vi "FeedbackDecode.vi"() -> ()   [LabVIEW 2020] (continued)
            n1857 = Cluster To Array(cluster=w1907) -> (array=w1906:bool[])
            n1858 = local read "DecodeClust"() -> (w1905:T5)
            n1859 = Boolean Array To Number(Boolean array=w1906) -> (number=w1904:u32)
            n1860 = local read "UEAHMIdx"() -> (w1924:i32[])
            n1861 = call "FeedbackDecode_PlotHeatmap.vi"("MousePos"=w1910, "Instance"=1, "Mode"=w1912) -> ("CurrPos"=w1923:i32)  [unwired: 3 in, 1 out]
            n1862 = call "FeedbackDecode_PlotHeatmap.vi"("MousePos"=w1911, "Instance"=0, "Mode"=w1912) -> ()  [unwired: 3 in, 2 out]
            n1863 = call "FeedbackDecode_PlotHeatmap.vi"("MousePos"=w1911, "Instance"=2, "Mode"=w1912) -> ()  [unwired: 3 in, 2 out]
            n1864 = Search 1D Array(1D array=w1924, element=w1923) -> (index of element=w1909:i32)  [unwired: 1 in]
            n1865 = Add(x=w1909, y=101) -> (x+y=w1903:i32)
            n1866 = case shown="4" w1904 {
              tunnel: w1903 -> [_ w1928 w1932]
              tunnel: w1905 -> [w1925 w1927 w1931]
              tunnel: [w1925 w1926 w1930] -> w1902
              frame 0, Default {
              }
              frame 18 {
                # "ctrl"
                n1867 = call "FeedbackDecode_UpdateDecodeClustElect.vi"("DecodeClustIn"=w1927, "KalmanElect"=w1928) -> ("DecodeClustOut"=w1926:T5)  [unwired: 1 in]
              }
              frame 4 {
                # "alt"
                n1868 = Unbundle By Name(w1931) -> ("BadUEAElects"=w1933:dbl[])
                n1869 = Insert Into Array(array=w1933, new element=w1932) -> (w1929:dbl[])  [unwired: 1 in]
                n1870 = Bundle By Name(cluster=w1931, "BadUEAElects"=w1929) -> (w1930:T5)
                n1871 = property on="BadUEAElects" class="Arr (strict)"("Val(Sgnl)"=w1929) -> ()  [unwired: 2 in, 2 out]
              }
            }
            n1872 = local read "LoopCnt"() -> (w1917:u64)
            n1873 = call-poly "FeedbackDecode_VariablesToString.vi"("Format"="%0.0f", "ValueIn"=w1903, "FieldName"="SelElect") -> ("StringOut"=w1919:string)  [unwired: 4 in]
            n1874 = local write "SelElect"(w1903) -> ()
            n1875 = local write "BaseCnt2"(w1917) -> ()
            n1876 = Bundle By Name(cluster=w1902, "ClearWfs"=TRUE, "SelElect"=w1903, "EventStr"=w1919) -> (w1901:T5)
            n1877 = call "FeedbackDecode_MLComCtrl.vi"("DecodeClustIn"=w1901, "Mode"=T19."SendEvent") -> ("DecodeClustOut"=w1900:T5)  [unwired: 6 in, 3 out]
            n1878 = local write "DecodeClust"(w1900) -> ()
          }
          event "EMGHM": Mouse Down {
            w1945 = cluster{"X":i32, "Y":i32} {"X"=0, "Y"=0} ("MousePos")
            w1946 = enum16{"Initialize", "Run", "Mouse"}."Mouse" ("Mode")
            n1879 = event-data() -> ("PlatMods"=w1942:T51, "Coords"=w1944:T45)  [unwired: 1 in, 4 out]
            n1880 = local read "DecodeClust"() -> (w1939:T5)
            n1881 = Cluster To Array(cluster=w1942) -> (array=w1941:bool[])
            n1882 = Boolean Array To Number(Boolean array=w1941) -> (number=w1940:u32)
            n1883 = local read "EMGHMIdx"() -> (w1958:i32[])
            n1884 = call "FeedbackDecode_PlotHeatmap.vi"("MousePos"=w1944, "Instance"=2, "Mode"=w1946) -> ("CurrPos"=w1957:i32)  [unwired: 3 in, 1 out]
            n1885 = call "FeedbackDecode_PlotHeatmap.vi"("MousePos"=w1945, "Instance"=0, "Mode"=w1946) -> ()  [unwired: 3 in, 2 out]
            n1886 = call "FeedbackDecode_PlotHeatmap.vi"("MousePos"=w1945, "Instance"=1, "Mode"=w1946) -> ()  [unwired: 3 in, 2 out]
            n1887 = Search 1D Array(1D array=w1958, element=w1957) -> (index of element=w1936:i32)  [unwired: 1 in]
            n1888 = Add(x=w1936, y=201) -> (x+y=w1938:i32)
            n1889 = case shown="4" w1940 {
              tunnel: w1938 -> [_ w1962 _]
              tunnel: w1939 -> [w1959 w1961 w1967]
              tunnel: [w1959 w1960 w1968] -> w1937
              tunnel: w1936 -> [_ _ w1969]
              frame 0, Default {
              }
              frame 18 {
                # "ctrl"
                n1890 = call "FeedbackDecode_UpdateDecodeClustElect.vi"("DecodeClustIn"=w1961, "KalmanElect"=w1962) -> ("DecodeClustOut"=w1960:T5)  [unwired: 1 in]
              }
              frame 4 {
                # "alt"
                n1891 = Quotient & Remainder(x=w1969, y=10.0) -> (x-y*floor(x/y)=w1973:dbl, floor(x/y)=w1975:dbl)
                n1892 = Increment(x=w1973) -> (x+1=w1974:dbl)
                n1893 = Multiply(x=w1975, y=4.0) -> (x*y=w1972:dbl)
                n1894 = Add(x=w1974, y=w1972) -> (x+y=w1963:dbl)
                n1895 = In Range and Coerce(upper limit=32.0, x=w1963, lower limit=1.0) -> (In Range?=w1964:bool)  [unwired: 1 out]
                n1896 = case shown="True" w1964 {
                  tunnel: w1963 -> [_ w1980]
                  tunnel: [w1976 w1979] -> w1968
                  tunnel: w1967 -> [w1976 w1977]
                  frame False {
                  }
                  frame True {
                    n1897 = Unbundle By Name(w1977) -> ("BadEMGChans"=w1981:dbl[])
                    n1898 = Insert Into Array(array=w1981, new element=w1980) -> (w1978:dbl[])  [unwired: 1 in]
                    n1899 = Bundle By Name(cluster=w1977, "BadEMGChans"=w1978) -> (w1979:T5)
                    n1900 = property on="BadEMGChans" class="Arr (strict)"("Val(Sgnl)"=w1978) -> ()  [unwired: 2 in, 2 out]
                  }
                }
              }
            }
            n1901 = call-poly "FeedbackDecode_VariablesToString.vi"("Format"="%0.0f", "ValueIn"=w1938, "FieldName"="SelElect") -> ("StringOut"=w1953:string)  [unwired: 4 in]
            n1902 = local write "SelElect"(w1938) -> ()
            n1903 = Bundle By Name(cluster=w1937, "ClearWfs"=TRUE, "SelElect"=w1938, "EventStr"=w1953) -> (w1934:T5)
            n1904 = local read "LoopCnt"() -> (w1951:u64)
            n1905 = call "FeedbackDecode_MLComCtrl.vi"("DecodeClustIn"=w1934, "Mode"=T19."SendEvent") -> ("DecodeClustOut"=w1935:T5)  [unwired: 6 in, 3 out]
            n1906 = local write "DecodeClust"(w1935) -> ()
            n1907 = local write "BaseCnt2"(w1951) -> ()
          }
          event Value Change {
            n1908 = event-data() -> ()  [unwired: 1 in, 6 out]
            n1909 = local read "EncodeClust"() -> (w1983:T9)
            n1910 = call "File Dialog2"("pattern (all files)"="StimParams*.txt") -> ("selected path"=w1986:path, "exists"=w1990:bool, "cancelled"=w1989:bool)  [unwired: 11 in, 1 out]
            n1911 = Unbundle By Name(w1983) -> ("SelPreset"=w1985:bool[], "Sel"=w1984:bool[])
            n1912 = local read "DecodeClust"() -> (w1982:T5)
            n1913 = Not(x=w1989) -> (.not. x?=w1991:bool)
            n1914 = And(x=w1990, y=w1991) -> (x .and. y?=w1987:bool)
            n1915 = case shown="True" w1987 {
              tunnel: w1986 -> [_ w2021]
              tunnel: w1985 -> [_ w2024]
              tunnel: w1984 -> [_ w2023]
              tunnel: w1983 -> [w1994 w2022]
              tunnel: w1982 -> [_ w2007]
              frame False {
                n1916 = Bundle By Name(cluster=w1994, "AdjClust.LoadTable"=FALSE) -> (w1993:T9)
                n1917 = local write "EncodeClust"(w1993) -> ()
              }
              frame True {
                n1918 = call-poly <vilib>:"Read Delimited Spreadsheet.vi"("file path (dialog if empty)"=w2021) -> ("all rows"=w2025:string[][])  [unwired: 9 in, 5 out]
                n1919 = Array Size(array=w2024) -> (size(s)=w2027:i32)
                n1920 = Array Size(array=w2023) -> (size(s)=w2030:i32)
                n1921 = Initialize Array(FALSE, w2027) -> (w2031:bool[])
                n1922 = Initialize Array(FALSE, w2030) -> (w2032:bool[])
                n1923 = Bundle By Name(cluster=w2022, "SelPreset"=w2031, "Sel"=w2032, "ParamsTable"=w2025, "AdjClust.LoadTable"=FALSE) -> (w2019:T9)
                n1924 = Path To String(path=w2021) -> (string=w2017:string)
                n1925 = call "FeedbackDecode_UpdateParamsTable.vi"("StimClustIn"=w2019) -> ("StimClustOut"=w2020:T9)  [unwired: 2 in]
                n1926 = call "FeedbackDecode_Params2UEA.vi"("StimClustIn"=w2020) -> ("StimClustOut"=w2002:T9)  [unwired: 2 in]
                n1927 = local read "LoopCnt"() -> (w2011:u64)
                n1928 = local read "NIPTime"() -> (w2000:dbl)
                n1929 = call "FeedbackDecode_BuildStimCmd.vi"("EncodeClustIn"=w2002) -> ("EncodeClustOut"=w2001:T9, "StimCmd"=w1996:string)  [unwired: 1 in]
                n1930 = Search and Replace String(input string=w2017, search string=":", replace string="@" ("replace string (\"\")")) -> (result string=w2004:string)  [unwired: 5 in, 3 out]
                n1931 = Format Into String(w2011) -> (resulting string=w2008:string)  [unwired: 3 in, 1 out]
                n1932 = call-poly "FeedbackDecode_VariablesToString.vi"("Format"="%0.0f", "ValueIn"=w2000, "FieldName"="NIPTime" ("Key Word")) -> ("StringOut"=w1997:string)  [unwired: 4 in]
                n1933 = local write "EncodeClust"(w2001) -> ()
                n1934 = Concatenate Strings("LoadStimParams:SS.EventID=" ("string"), w2008) -> (w2010:string)
                n1935 = Concatenate Strings(w2010, ";", "SS.StimParamsFile='" ("string"), w2004, "';" ("string"), w1996, w1997) -> (w2006:string)
                n1936 = local write "StimCmd"(w1996) -> ()
                n1937 = Bundle By Name(cluster=w2007, "EventStr"=w2006) -> (w2009:T5)
                n1938 = local read "EventParamsFID"() -> (w2015:refnum<file>)
                n1939 = call "FeedbackDecode_MLComCtrl.vi"("DecodeClustIn"=w2009, "Mode"=T19."SendEvent") -> ()  [unwired: 6 in, 4 out]
                n1940 = call "FeedbackDecode_WriteTextEOL.vi"("text"=w2006, "refnum in"=w2015) -> ()  [unwired: 8 in, 2 out]
              }
            }
          }
          event Value Change {
            n1941 = event-data() -> ()  [unwired: 1 in, 6 out]
            n1942 = local read "EncodeClust"() -> (w2034:T9)
            n1943 = call "File Dialog3"("pattern (all files)"="StimPresets*.txt") -> ("selected path"=w2037:path, "exists"=w2041:bool, "cancelled"=w2040:bool)  [unwired: 11 in, 1 out]
            n1944 = Unbundle By Name(w2034) -> ("SelPreset"=w2036:bool[], "Sel"=w2035:bool[])
            n1945 = local read "DecodeClust"() -> (w2033:T5)
            n1946 = Not(x=w2040) -> (.not. x?=w2042:bool)
            n1947 = And(x=w2041, y=w2042) -> (x .and. y?=w2038:bool)
            n1948 = case shown="True" w2038 {
              tunnel: w2037 -> [_ w2073]
              tunnel: w2036 -> [_ w2076]
              tunnel: w2035 -> [_ w2075]
              tunnel: w2034 -> [w2045 w2074]
              tunnel: w2033 -> [_ w2060]
              frame False {
                n1949 = Bundle By Name(cluster=w2045, "AdjClust.LoadTable"=FALSE) -> (w2044:T9)
                n1950 = local write "EncodeClust"(w2044) -> ()
              }
              frame True {
                n1951 = call-poly <vilib>:"Read Delimited Spreadsheet.vi"("file path (dialog if empty)"=w2073) -> ("all rows"=w2077:string[][])  [unwired: 9 in, 5 out]
                n1952 = Array Size(array=w2076) -> (size(s)=w2079:i32)
                n1953 = Array Size(array=w2075) -> (size(s)=w2082:i32)
                n1954 = Initialize Array(FALSE, w2079) -> (w2083:bool[])
                n1955 = Initialize Array(FALSE, w2082) -> (w2084:bool[])
                n1956 = Bundle By Name(cluster=w2074, "SelPreset"=w2083, "Sel"=w2084, "PresetTable"=w2077, "PresetClust.Load"=FALSE ("AdjClust.LoadTable")) -> (w2048:T9)
                n1957 = Path To String(path=w2073) -> (string=w2070:string)
                n1958 = call "FeedbackDecode_UpdatePresetsTable.vi"("StimClustIn"=w2048) -> ("StimClustOut"=w2047:T9)  [unwired: 2 in]
                n1959 = call "FeedbackDecode_UpdateParamsTable.vi"("StimClustIn"=w2047) -> ("StimClustOut"=w2072:T9)  [unwired: 2 in]
                n1960 = call "FeedbackDecode_Params2UEA.vi"("StimClustIn"=w2072) -> ("StimClustOut"=w2055:T9)  [unwired: 2 in]
                n1961 = local read "LoopCnt"() -> (w2064:u64)
                n1962 = local read "NIPTime"() -> (w2053:dbl)
                n1963 = call "FeedbackDecode_BuildStimCmd.vi"("EncodeClustIn"=w2055) -> ("EncodeClustOut"=w2054:T9, "StimCmd"=w2049:string)  [unwired: 1 in]
                n1964 = Search and Replace String(input string=w2070, search string=":", replace string="@" ("replace string (\"\")")) -> (result string=w2057:string)  [unwired: 5 in, 3 out]
                n1965 = Format Into String(w2064) -> (resulting string=w2061:string)  [unwired: 3 in, 1 out]
                n1966 = call-poly "FeedbackDecode_VariablesToString.vi"("Format"="%0.0f", "ValueIn"=w2053, "FieldName"="NIPTime" ("Key Word")) -> ("StringOut"=w2050:string)  [unwired: 4 in]
                n1967 = local write "EncodeClust"(w2054) -> ()
                n1968 = Concatenate Strings("LoadPresets:SS.EventID=" ("string"), w2061) -> (w2063:string)
                n1969 = Concatenate Strings(w2063, ";", "SS.PresetsFile='" ("string"), w2057, "';" ("string"), w2049, w2050) -> (w2059:string)
                n1970 = local write "StimCmd"(w2049) -> ()
                n1971 = Bundle By Name(cluster=w2060, "EventStr"=w2059) -> (w2062:T5)
                n1972 = local read "EventParamsFID"() -> (w2068:refnum<file>)
                n1973 = call "FeedbackDecode_MLComCtrl.vi"("DecodeClustIn"=w2062, "Mode"=T19."SendEvent") -> ()  [unwired: 6 in, 4 out]
                n1974 = call "FeedbackDecode_WriteTextEOL.vi"("text"=w2059, "refnum in"=w2068) -> ()  [unwired: 8 in, 2 out]
              }
            }
          }
          event Value Change {
            n1975 = event-data() -> ()  [unwired: 1 in, 6 out]
            n1976 = local read "DataPath"() -> (w2089:path)
            n1977 = call "File Dialog"("start path"=w2089) -> ("selected path"=w2086:path, "cancelled"=w2088:bool)  [unwired: 11 in, 2 out]
            n1978 = local read "EncodeClust"() -> (w2087:T9)
            n1979 = local read "DecodeClust"() -> (w2085:T5)
            n1980 = case shown="False" w2088 {
              tunnel: w2087 -> [w2100 w2127]
              tunnel: w2086 -> [w2101 _]
              tunnel: w2085 -> [w2091 _]
              frame False {
                w2110 = "_" ("string")
                n1981 = Strip Path(path=w2101) -> (stripped path=w2108:path, name=w2109:string)
                n1982 = Unbundle By Name(w2091) -> ("DataFolder"=w2098:string)
                n1983 = Get Date/Time In Seconds() -> (seconds since 1Jan1904=w2104:timestamp)
                n1984 = Format Date/Time String(time format string (%c)="%H%M%S", seconds (now)=w2104) -> (date/time string=w2106:string)  [unwired: 1 in]
                n1985 = Concatenate Strings("StimParams_" ("name or relative path"), w2098, w2110, w2109, w2110, w2106, ".txt" ("string")) -> (w2107:string)
                n1986 = Unbundle By Name(w2100) -> ("ParamsTable"=w2102:string[][])
                n1987 = Bundle By Name(cluster=w2100, "AdjClust.SaveTable"=FALSE ("Save")) -> (w2120:T9)
                n1988 = Build Path(base path=w2108, name or relative path=w2107) -> (appended path=w2111:path)
                n1989 = call-poly <vilib>:"Write Delimited Spreadsheet.vi"("file path (dialog if empty)"=w2111, "2D data"=w2102) -> ()  [unwired: 12 in, 2 out]
                n1990 = Path To String(path=w2111) -> (string=w2095:string)
                n1991 = local read "LoopCnt"() -> (w2123:u64)
                n1992 = local write "EncodeClust"(w2120) -> ()
                n1993 = Format Into String(w2123) -> (resulting string=w2112:string)  [unwired: 3 in, 1 out]
                n1994 = Search and Replace String(input string=w2095, search string=":", replace string="@" ("replace string (\"\")")) -> (result string=w2093:string)  [unwired: 5 in, 3 out]
                n1995 = local read "NIPTime"() -> (w2117:dbl)
                n1996 = Concatenate Strings("SaveStimParams:SS.EventID=" ("string"), w2112, ";") -> (w2118:string)
                n1997 = local read "EventParamsFID"() -> (w2126:refnum<file>)
                n1998 = call-poly "FeedbackDecode_VariablesToString.vi"("Format"="%0.0f", "ValueIn"=w2117, "FieldName"="NIPTime" ("Key Word")) -> ("StringOut"=w2114:string)  [unwired: 4 in]
                n1999 = Concatenate Strings(w2118, "SS.StimParamsFile='" ("string"), w2093, "';" ("string"), w2114) -> (w2113:string)
                n2000 = call "FeedbackDecode_WriteTextEOL.vi"("text"=w2113, "refnum in"=w2126) -> ()  [unwired: 8 in, 2 out]
                n2001 = Bundle By Name(cluster=w2091, "EventStr"=w2113) -> (w2122:T5)
                n2002 = call "FeedbackDecode_MLComCtrl.vi"("DecodeClustIn"=w2122, "Mode"=T19."SendEvent") -> ()  [unwired: 6 in, 4 out]
              }
              frame True {
                n2003 = Bundle By Name(cluster=w2127, "AdjClust.SaveTable"=FALSE ("Save")) -> (w2129:T9)
                n2004 = local write "EncodeClust"(w2129) -> ()
              }
            }
          }
          event Value Change {
            n2005 = event-data() -> ()  [unwired: 1 in, 6 out]
            n2006 = local read "DataPath"() -> (w2134:path)
            n2007 = call "File Dialog4"("start path"=w2134) -> ("selected path"=w2131:path, "cancelled"=w2133:bool)  [unwired: 11 in, 2 out]
            n2008 = local read "EncodeClust"() -> (w2132:T9)
            n2009 = local read "DecodeClust"() -> (w2130:T5)
            n2010 = case shown="False" w2133 {
              tunnel: w2132 -> [w2145 w2172]
              tunnel: w2131 -> [w2146 _]
              tunnel: w2130 -> [w2136 _]
              frame False {
                w2155 = "_" ("string")
                n2011 = Strip Path(path=w2146) -> (stripped path=w2153:path, name=w2154:string)
                n2012 = Unbundle By Name(w2136) -> ("DataFolder"=w2143:string)
                n2013 = Get Date/Time In Seconds() -> (seconds since 1Jan1904=w2149:timestamp)
                n2014 = Format Date/Time String(time format string (%c)="%H%M%S", seconds (now)=w2149) -> (date/time string=w2151:string)  [unwired: 1 in]
                n2015 = Concatenate Strings("StimPresets_" ("name or relative path"), w2143, w2155, w2154, w2155, w2151, ".txt" ("string")) -> (w2152:string)
                n2016 = Unbundle By Name(w2145) -> ("PresetTable"=w2147:string[][])
                n2017 = Build Path(base path=w2153, name or relative path=w2152) -> (appended path=w2156:path)
                n2018 = Bundle By Name(cluster=w2145, "PresetClust.Save"=FALSE ("Save")) -> (w2165:T9)
                n2019 = call-poly <vilib>:"Write Delimited Spreadsheet.vi"("file path (dialog if empty)"=w2156, "2D data"=w2147) -> ()  [unwired: 12 in, 2 out]
                n2020 = Path To String(path=w2156) -> (string=w2140:string)
                n2021 = local read "LoopCnt"() -> (w2168:u64)
                n2022 = local write "EncodeClust"(w2165) -> ()
                n2023 = Format Into String(w2168) -> (resulting string=w2157:string)  [unwired: 3 in, 1 out]
                n2024 = Search and Replace String(input string=w2140, search string=":", replace string="@" ("replace string (\"\")")) -> (result string=w2138:string)  [unwired: 5 in, 3 out]
                n2025 = local read "NIPTime"() -> (w2162:dbl)
                n2026 = Concatenate Strings("SavePresets:SS.EventID=" ("string"), w2157, ";") -> (w2163:string)
                n2027 = local read "EventParamsFID"() -> (w2171:refnum<file>)
                n2028 = call-poly "FeedbackDecode_VariablesToString.vi"("Format"="%0.0f", "ValueIn"=w2162, "FieldName"="NIPTime" ("Key Word")) -> ("StringOut"=w2159:string)  [unwired: 4 in]
                n2029 = Concatenate Strings(w2163, "SS.PresetsFile='" ("string"), w2138, "';" ("string"), w2159) -> (w2158:string)
                n2030 = call "FeedbackDecode_WriteTextEOL.vi"("text"=w2158, "refnum in"=w2171) -> ()  [unwired: 8 in, 2 out]
                n2031 = Bundle By Name(cluster=w2136, "EventStr"=w2158) -> (w2167:T5)
                n2032 = call "FeedbackDecode_MLComCtrl.vi"("DecodeClustIn"=w2167, "Mode"=T19."SendEvent") -> ()  [unwired: 6 in, 4 out]
              }
              frame True {
                n2033 = Bundle By Name(cluster=w2172, "AdjClust.SaveTable"=FALSE ("Save")) -> (w2174:T9)
                n2034 = local write "EncodeClust"(w2174) -> ()
              }
            }
          }
          event Value Change {
            n2035 = event-data() -> ()  [unwired: 1 in, 6 out]
            n2036 = local read "EncodeClust"() -> (w2179:T9)
            n2037 = call "FeedbackDecode_Params2Preset.vi"("StimClustIn"=w2179) -> ("StimClustOut"=w2178:T9)  [unwired: 2 in]
            n2038 = local read "LoopCnt"() -> (w2188:u64)
            n2039 = call "FeedbackDecode_UpdateParamsTable.vi"("StimClustIn"=w2178) -> ("StimClustOut"=w2177:T9)  [unwired: 2 in]
            n2040 = call "FeedbackDecode_Params2UEA.vi"("StimClustIn"=w2177) -> ("StimClustOut"=w2176:T9)  [unwired: 2 in]
            n2041 = Format Into String(w2188) -> (resulting string=w2180:string)  [unwired: 3 in, 1 out]
            n2042 = local read "NIPTime"() -> (w2184:dbl)
            n2043 = call "FeedbackDecode_BuildStimCmd.vi"("EncodeClustIn"=w2176) -> ("EncodeClustOut"=w2194:T9, "StimCmd"=w2175:string)  [unwired: 1 in]
            n2044 = local read "EventParamsFID"() -> (w2192:refnum<file>)
            n2045 = Concatenate Strings("UpdateStim:SS.EventID=" ("string"), w2180) -> (w2187:string)
            n2046 = call-poly "FeedbackDecode_VariablesToString.vi"("Format"="%0.0f", "ValueIn"=w2184, "FieldName"="NIPTime" ("Key Word")) -> ("StringOut"=w2181:string)  [unwired: 4 in]
            n2047 = local read "DecodeClust"() -> (w2193:T5)
            n2048 = Concatenate Strings(w2187, ";", w2175, w2181) -> (w2186:string)
            n2049 = call "FeedbackDecode_WriteTextEOL.vi"("text"=w2186, "refnum in"=w2192) -> ()  [unwired: 8 in, 2 out]
            n2050 = Bundle By Name(cluster=w2193, "EventStr"=w2186) -> (w2185:T5)
            n2051 = local write "StimCmd"(w2175) -> ()
            n2052 = local write "EncodeClust"(w2194) -> ()
            n2053 = call "FeedbackDecode_MLComCtrl.vi"("DecodeClustIn"=w2185, "Mode"=T19."SendEvent") -> ()  [unwired: 6 in, 4 out]
          }
          event Value Change {
            n2054 = event-data() -> ("NewVal"=w2201:bool[], "OldVal"=w2200:bool[])  [unwired: 1 in, 4 out]
            n2055 = call "FeedbackDecode_UpdateSelPresets.vi"("OldSelIn"=w2200, "NewSelIn"=w2201) -> ("OldSelOut"=w2199:bool[], "NewSelOut"=w2198:bool[])
            n2056 = Exclusive Or(1:w2199, 2:w2198) -> (0:w2196:bool[])
            n2057 = Or Array Elements(Boolean array=w2198) -> (logical OR=w2197:bool)
            n2058 = case shown="False" w2197 {
              tunnel: w2196 -> [w2205 _]
              frame True {
                n2059 = local read "EncodeClust"() -> (w2206:T9)
                n2060 = Bundle By Name(cluster=w2206, "SelPreset"=w2205) -> (w2204:T9)
                n2061 = call "FeedbackDecode_UpdatePresetsTable.vi"("StimClustIn"=w2204) -> ("StimClustOut"=w2209:T9)  [unwired: 2 in]
                n2062 = local read "LoopCnt"() -> (w2218:u64)
                n2063 = call "FeedbackDecode_UpdateParamsTable.vi"("StimClustIn"=w2209) -> ("StimClustOut"=w2208:T9)  [unwired: 2 in]
                n2064 = call "FeedbackDecode_Params2UEA.vi"("StimClustIn"=w2208) -> ("StimClustOut"=w2207:T9)  [unwired: 2 in]
                n2065 = Format Into String(w2218) -> (resulting string=w2210:string)  [unwired: 3 in, 1 out]
                n2066 = local read "NIPTime"() -> (w2214:dbl)
                n2067 = call "FeedbackDecode_BuildStimCmd.vi"("EncodeClustIn"=w2207) -> ("EncodeClustOut"=w2224:T9, "StimCmd"=w2203:string)  [unwired: 1 in]
                n2068 = local read "EventParamsFID"() -> (w2222:refnum<file>)
                n2069 = Concatenate Strings("UpdateStim:SS.EventID=" ("string"), w2210) -> (w2217:string)
                n2070 = call-poly "FeedbackDecode_VariablesToString.vi"("Format"="%0.0f", "ValueIn"=w2214, "FieldName"="NIPTime" ("Key Word")) -> ("StringOut"=w2211:string)  [unwired: 4 in]
                n2071 = local read "DecodeClust"() -> (w2223:T5)
                n2072 = Concatenate Strings(w2217, ";", w2203, w2211) -> (w2216:string)
                n2073 = call "FeedbackDecode_WriteTextEOL.vi"("text"=w2216, "refnum in"=w2222) -> ()  [unwired: 8 in, 2 out]
                n2074 = Bundle By Name(cluster=w2223, "EventStr"=w2216) -> (w2215:T5)
                n2075 = local write "StimCmd"(w2203) -> ()
                n2076 = local write "EncodeClust"(w2224) -> ()
                n2077 = call "FeedbackDecode_MLComCtrl.vi"("DecodeClustIn"=w2215, "Mode"=T19."SendEvent") -> ()  [unwired: 6 in, 4 out]
              }
              frame False {
                n2078 = local read "EncodeClust"() -> (w2227:T9)
                n2079 = Unbundle By Name(w2227) -> ("Sel"=w2229:bool[])
                n2080 = Array Size(array=w2229) -> (size(s)=w2230:i32)
                n2081 = Initialize Array(FALSE, w2230) -> (w2228:bool[])
                n2082 = Bundle By Name(cluster=w2227, "Sel"=w2228) -> (w2226:T9)
                n2083 = local read "LoopCnt"() -> (w2242:u64)
                n2084 = call "FeedbackDecode_UpdateParamsTable.vi"("StimClustIn"=w2226) -> ("StimClustOut"=w2233:T9)  [unwired: 2 in]
                n2085 = call "FeedbackDecode_Params2UEA.vi"("StimClustIn"=w2233) -> ("StimClustOut"=w2232:T9)  [unwired: 2 in]
                n2086 = Format Into String(w2242) -> (resulting string=w2234:string)  [unwired: 3 in, 1 out]
                n2087 = local read "NIPTime"() -> (w2238:dbl)
                n2088 = call "FeedbackDecode_BuildStimCmd.vi"("EncodeClustIn"=w2232) -> ("EncodeClustOut"=w2248:T9, "StimCmd"=w2225:string)  [unwired: 1 in]
                n2089 = local read "EventParamsFID"() -> (w2246:refnum<file>)
                n2090 = Concatenate Strings("UpdateStim:SS.EventID=" ("string"), w2234) -> (w2241:string)
                n2091 = call-poly "FeedbackDecode_VariablesToString.vi"("Format"="%0.0f", "ValueIn"=w2238, "FieldName"="NIPTime" ("Key Word")) -> ("StringOut"=w2235:string)  [unwired: 4 in]
                n2092 = local read "DecodeClust"() -> (w2247:T5)
                n2093 = Concatenate Strings(w2241, ";", w2225, w2235) -> (w2240:string)
                n2094 = call "FeedbackDecode_WriteTextEOL.vi"("text"=w2240, "refnum in"=w2246) -> ()  [unwired: 8 in, 2 out]
                n2095 = Bundle By Name(cluster=w2247, "EventStr"=w2240) -> (w2239:T5)
                n2096 = local write "StimCmd"(w2225) -> ()
                n2097 = local write "EncodeClust"(w2248) -> ()
                n2098 = call "FeedbackDecode_MLComCtrl.vi"("DecodeClustIn"=w2239, "Mode"=T19."SendEvent") -> ()  [unwired: 6 in, 4 out]
              }
            }
          }
          event Value Change {
            n2099 = event-data() -> ()  [unwired: 1 in, 6 out]
            n2100 = local read "EncodeClust"() -> (w2253:T9)
            n2101 = call "FeedbackDecode_UEA2Params.vi"("StimClustIn"=w2253) -> ("StimClustOut"=w2252:T9)  [unwired: 2 in]
            n2102 = local read "LoopCnt"() -> (w2262:u64)
            n2103 = call "FeedbackDecode_UpdateParamsTable.vi"("StimClustIn"=w2252) -> ("StimClustOut"=w2251:T9)  [unwired: 2 in]
            n2104 = call "FeedbackDecode_Params2Preset.vi"("StimClustIn"=w2251) -> ("StimClustOut"=w2250:T9)  [unwired: 2 in]
            n2105 = Format Into String(w2262) -> (resulting string=w2254:string)  [unwired: 3 in, 1 out]
            n2106 = local read "NIPTime"() -> (w2258:dbl)
            n2107 = call "FeedbackDecode_BuildStimCmd.vi"("EncodeClustIn"=w2250) -> ("EncodeClustOut"=w2268:T9, "StimCmd"=w2249:string)  [unwired: 1 in]
            n2108 = local read "EventParamsFID"() -> (w2266:refnum<file>)
            n2109 = Concatenate Strings("UpdateStim:SS.EventID=" ("string"), w2254) -> (w2261:string)
            n2110 = call-poly "FeedbackDecode_VariablesToString.vi"("Format"="%0.0f", "ValueIn"=w2258, "FieldName"="NIPTime" ("Key Word")) -> ("StringOut"=w2255:string)  [unwired: 4 in]
            n2111 = local read "DecodeClust"() -> (w2267:T5)
            n2112 = Concatenate Strings(w2261, ";", w2249, w2255) -> (w2260:string)
            n2113 = call "FeedbackDecode_WriteTextEOL.vi"("text"=w2260, "refnum in"=w2266) -> ()  [unwired: 8 in, 2 out]
            n2114 = Bundle By Name(cluster=w2267, "EventStr"=w2260) -> (w2259:T5)
            n2115 = local write "StimCmd"(w2249) -> ()
            n2116 = local write "EncodeClust"(w2268) -> ()
            n2117 = call "FeedbackDecode_MLComCtrl.vi"("DecodeClustIn"=w2259, "Mode"=T19."SendEvent") -> ()  [unwired: 6 in, 4 out]
          }
          event Value Change {
            n2118 = event-data() -> ()  [unwired: 1 in, 6 out]
            n2119 = local read "EncodeClust"() -> (w2275:T9)
            n2120 = call "FeedbackDecode_AdjParamsTable.vi"("StimClustIn"=w2275, "Mode"=enum16{"Set", "Add", "Sub"}."Set") -> ("StimClustOut"=w2273:T9)  [unwired: 1 in]
            n2121 = Bundle By Name(cluster=w2273, "AdjClust.Set"=FALSE) -> (w2271:T9)
            n2122 = local read "LoopCnt"() -> (w2285:u64)
            n2123 = call "FeedbackDecode_Params2Preset.vi"("StimClustIn"=w2271) -> ("StimClustOut"=w2276:T9)  [unwired: 2 in]
            n2124 = Format Into String(w2285) -> (resulting string=w2277:string)  [unwired: 3 in, 1 out]
            n2125 = local read "NIPTime"() -> (w2281:dbl)
            n2126 = call "FeedbackDecode_BuildStimCmd.vi"("EncodeClustIn"=w2276) -> ("EncodeClustOut"=w2291:T9, "StimCmd"=w2270:string)  [unwired: 1 in]
            n2127 = local read "EventParamsFID"() -> (w2289:refnum<file>)
            n2128 = Concatenate Strings("UpdateStim:SS.EventID=" ("string"), w2277) -> (w2284:string)
            n2129 = call-poly "FeedbackDecode_VariablesToString.vi"("Format"="%0.0f", "ValueIn"=w2281, "FieldName"="NIPTime" ("Key Word")) -> ("StringOut"=w2278:string)  [unwired: 4 in]
            n2130 = local read "DecodeClust"() -> (w2290:T5)
            n2131 = Concatenate Strings(w2284, ";", w2270, w2278) -> (w2283:string)
            n2132 = call "FeedbackDecode_WriteTextEOL.vi"("text"=w2283, "refnum in"=w2289) -> ()  [unwired: 8 in, 2 out]
            n2133 = Bundle By Name(cluster=w2290, "EventStr"=w2283) -> (w2282:T5)
            n2134 = local write "StimCmd"(w2270) -> ()
            n2135 = local write "EncodeClust"(w2291) -> ()
